vi "Serializer_Test.vi"() -> ()   [LabVIEW 2013]
uses:
  source/Serializer/Serializer.lvclass
panel:
  in  "Type Cast":bool
  out "error out":errorcluster
  out "Variant":variant
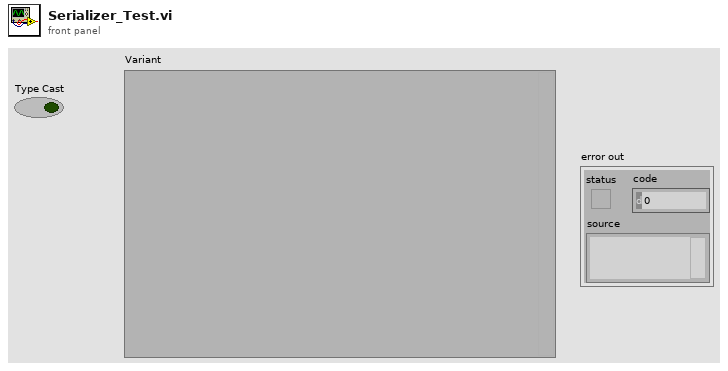
[diagram p1: front panel]
types:
  T1 = cluster{"Numeric":dbl, "Configuration Path":path, "Referenced?":bool, "Attribute":string}
  T2 = cluster{"Number1":dbl, "MyPath":path, "Initialized?":bool, "MyString with Spaces":string}
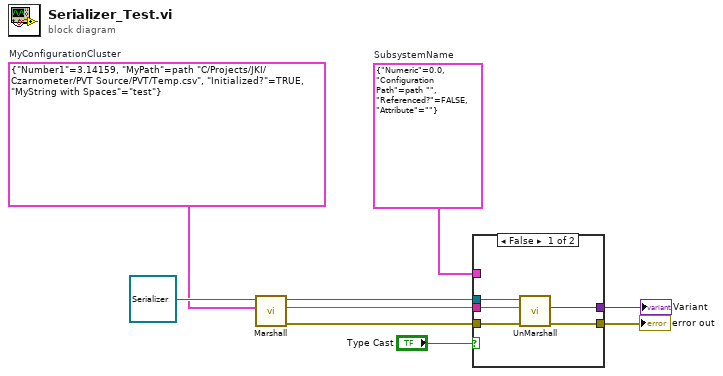
[diagram p0: block diagram]
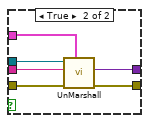
[diagram p2: hidden frame]
diagram:
  w2 = T1 {"Numeric"=0.0, "Configuration Path"=path "", "Referenced?"=FALSE, "Attribute"=""}  # SubsystemName
  w6 = T2 {"Number1"=3.14159, "MyPath"=path "C:/Projects/JKI/Czarnometer/PVT Source/PVT/Temp.csv", "Initialized?"=TRUE, "MyString with Spaces"="test"}  # MyConfigurationCluster
  n1 = call-dynamic "Marshall.vi"("Variant"=w6, "Serializer in"=refnum<class "Serializer.lvclass"> refnum) -> ("error out"=w4:errorcluster, "String"=w7:string, "Serializer out"=w8:refnum<class "Serializer.lvclass">)  [unwired: 7 in]
  n2 = case shown="False" "Type Cast" {
    tunnel: w8 -> [w14 w20]
    tunnel: w7 -> [w12 w19]
    tunnel: [w10 w18] -> w5
    tunnel: w4 -> [w13 w17]
    tunnel: [w11 w16] -> w3
    tunnel: w2 -> [_ w15]
    frame False {
      n3 = call-dynamic "UnMarshall.vi"("error in (no error)"=w13, "String"=w12, "Serializer in"=w14) -> ("error out"=w11:errorcluster, "Variant"=w10:variant)  [unwired: 6 in, 1 out]
    }
    frame True {
      n4 = call-dynamic "UnMarshall.vi"("Type"=w15, "error in (no error)"=w17, "String"=w19, "Serializer in"=w20) -> ("error out"=w16:errorcluster, "Variant"=w18:variant)  [unwired: 5 in, 1 out]
    }
  }
  "Variant" <- w5
  "error out" <- w3
